vi "RTS APLUS Points.vi"(7 "Point Data":T1[](array[typedef]), 8 "Error In":errorcluster, 11 "APLUS Data":string[](array[string])) -> (0 "Error Out":errorcluster, 3 "APLUS Data":T2[](array[typedef]))   [LabVIEW 2018]
uses:
  Washer DOE/Type Definitions/DOE Data Save Modifier.ctl
  Type Definitions/RTS Point File.ctl
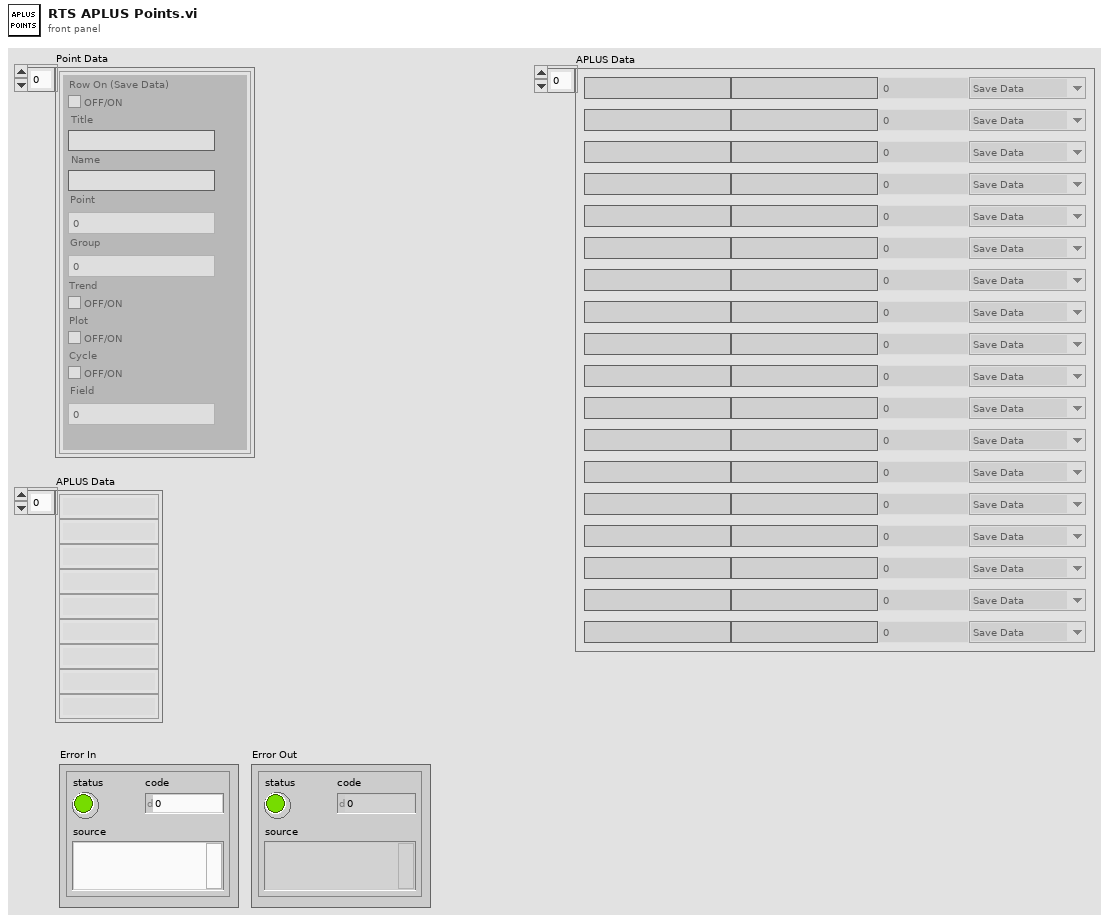
[diagram p1: front panel]
types:
  T1 = typedef "RTS Point File.ctl" = cluster{"Title":string, "Name":string, "Point":u8, "Plot":bool, "Trend":bool, "Cycle":bool, "Field":u8, "Row On (Save Data)":bool, "Group":u8}
  T2 = typedef "DOE Data Save Modifier.ctl" = cluster{"Name":string, "Title":string, "Save Status":enum16{"Save Data", "Don't Save Data"}, "Group":u8, "Field":u8}
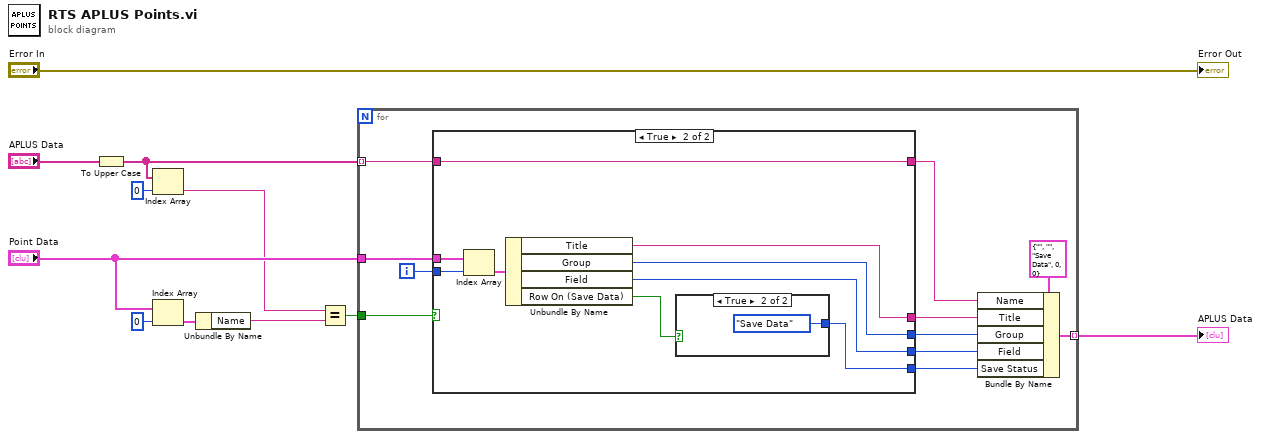
[diagram p0: block diagram]
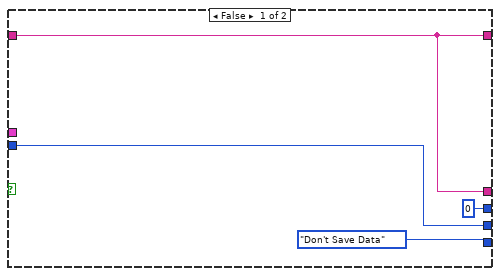
[diagram p2: hidden frame]
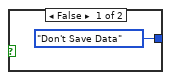
[diagram p3: hidden frame]
diagram:
  n1 = To Upper Case(1:"APLUS Data") -> (0:w2:string[])
  n2 = Index Array(array=w2, index=0) -> (element=w1:string)
  n3 = Index Array(array="Point Data", index=0) -> (element=w6:T1)
  n4 = Unbundle By Name(w6) -> ("Name"=w5:string)
  n5 = Equal?(x=w1, y=w5) -> (x = y?=w4:bool)
  n6 = for {
    tunnel: "Point Data" -> [w17]
    tunnel: [w19] -> w11 mode=indexing
    tunnel: w2 -> [w13] mode=indexing
    tunnel: w4 -> [w14]
    i -> [w16]
    n7 = case shown="True" w14 {
      tunnel: [w25 w35] -> w21
      tunnel: [u8 0 ("Group") w34] -> w20
      tunnel: [w23 w33] -> w18
      tunnel: w17 -> [_ w32]
      tunnel: w16 -> [w23 w31]
      tunnel: [enum16{"Save Data", "Don't Save Data"}."Don't Save Data" ("Save Status") w28] -> w15
      tunnel: w13 -> [w25 w27]
      tunnel: [w25 w27] -> w12
      frame False {
      }
      frame True {
        n8 = Index Array(array=w32, index=w31) -> (element=w30:T1)
        n9 = Unbundle By Name(w30) -> ("Title"=w35:string, "Group"=w34:u8, "Field"=w33:u8, "Row On (Save Data)"=w29:bool)
        n10 = case shown="True" w29 {
          tunnel: [enum16{"Save Data", "Don't Save Data"}."Don't Save Data" ("Save Status") enum16{"Save Data", "Don't Save Data"}."Save Data" ("Save Status")] -> w28
          frame False {
          }
          frame True {
          }
        }
      }
    }
    n11 = Bundle By Name(cluster=T2 {"Name"="", "Title"="", "Save Status"=enum."Save Data", "Group"=0, "Field"=0} ("Cluster"), "Name"=w12, "Title"=w21, "Group"=w20, "Field"=w18, "Save Status"=w15) -> (w19:T2)
  }
  "APLUS Data" <- w11
  "Error Out" <- "Error In"
